vi "Save-Recall Setup.vi"(8 "error in (no error)":errorcluster, 9 "Memory Address (1)":i32=1, 10 "Action (0:Save)":u16(ring) items=["Save", "Recall"], 11 "VISA resource name":refnum<visa-resource-name>) -> (0 "error out":errorcluster, 3 "VISA resource name out":refnum<visa-resource-name>)   [LabVIEW 2015, in "Agilent E363X Series.lvlib"]
doc: "Allows users to save or recall the operating state of the power supply to 3 memory locations in non-volatile memory."
uses:
  <instrlib>/Agilent E363X Series/Agilent E363X Series.lvlib
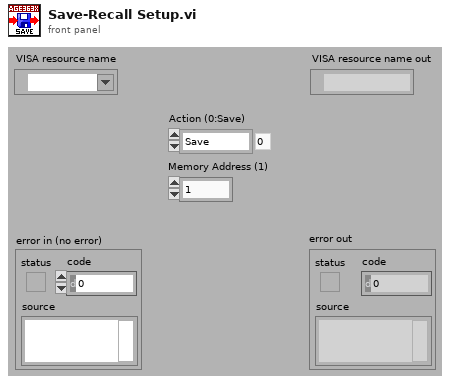
[diagram p1: front panel]
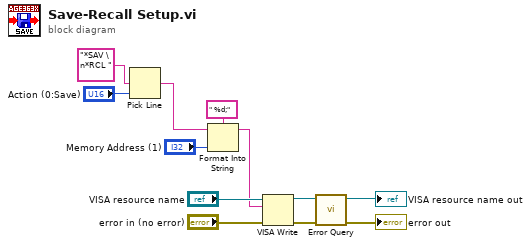
[diagram p0: block diagram]
diagram:
  n1 = Pick Line(multi-line string="*SAV \n*RCL ", line index="Action (0:Save)") -> (output string=w4:string)  [unwired: 1 in]
  n2 = Format Into String(format string=" %d;", initial string=w4, "Memory Address (1)") -> (resulting string=w3:string)  [unwired: 1 in, 1 out]
  n3 = VISA Write(VISA resource name="VISA resource name", write buffer=w3, error in (no error)="error in (no error)") -> (VISA resource name out=w8:refnum<visa-resource-name>, error out=w7:errorcluster)  [unwired: 1 out]
  n4 = call <instrlib>:"Error Query.vi"("error in (no error)"=w7, "VISA resource name"=w8) -> ("error out"=→"error out":errorcluster, "VISA resource name out"=→"VISA resource name out":refnum<visa-resource-name>)  [unwired: 6 in, 2 out]
